vi "Average Single Triggers.vi"(8 "error in (no error)":errorcluster, 9 "Average Count (1)":i32=10, 11 "VISA session":refnum<visa-resource-name>) -> (0 "error out":errorcluster, 3 "VISA session out":refnum<visa-resource-name>)   [LabVIEW 2019]
doc: "Very simple (non-optimized) way to get just enough triggers to average the specified amount."
panel:
  out "i":i32
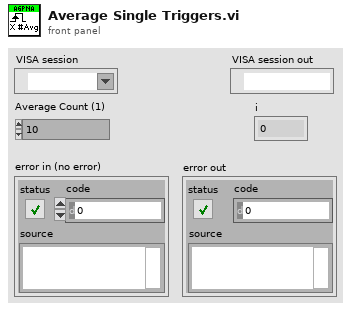
[diagram p1: front panel]
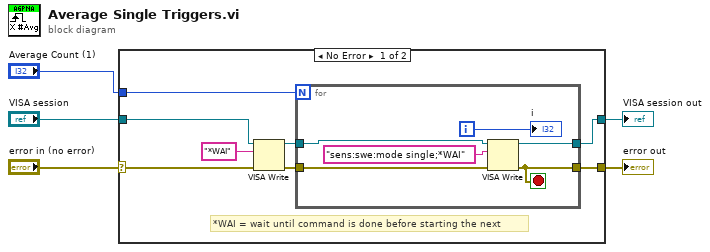
[diagram p0: block diagram]
diagram:
  n1 = case shown="No Error" "error in (no error)" {
    selector: "error in (no error)" -> [w6 w21]
    tunnel: "Average Count (1)" -> [w13 _]
    tunnel: "VISA session" -> [w10 w20]
    tunnel: [w12 w21] -> w2
    tunnel: [w11 w20] -> w1
    frame No Error {
      # "*WAI = wait until command is done before starting the next"
      n2 = VISA Write(VISA resource name=w10, write buffer="*WAI" ("Command"), error in (no error)=w6) -> (VISA resource name out=w9:refnum<visa-resource-name>, error out=w7:errorcluster)  [unwired: 1 out]
      n3 = for {
        N: w13 -> [_]
        tunnel: [w18] -> w12
        tunnel: w9 -> [w16]
        tunnel: [w15] -> w11
        tunnel: w7 -> [w14]
        i -> [w17]
        stop <- w18 stop-if-true
        n4 = VISA Write(VISA resource name=w16, write buffer="sens:swe:mode single;*WAI", error in (no error)=w14) -> (VISA resource name out=w15:refnum<visa-resource-name>, error out=w18:errorcluster)  [unwired: 1 out]
        "i" <- w17
      }
    }
    frame Error {
    }
  }
  "VISA session out" <- w1
  "error out" <- w2
